vi "Get Debugger.vi"(8 "error in (no error)":errorcluster, 11 "Main In":refnum<class "Main.lvclass">) -> (0 "error out":errorcluster, 2 "Debugger.lvclass":refnum<class "Debugger.lvclass">, 3 "Main Out":refnum<class "Main.lvclass">)   [LabVIEW 2020, in "Main.lvclass"]
uses:
  Main.lvclass
  Debugger/Debugger.lvclass
  Main.lvclass/Main.ctl
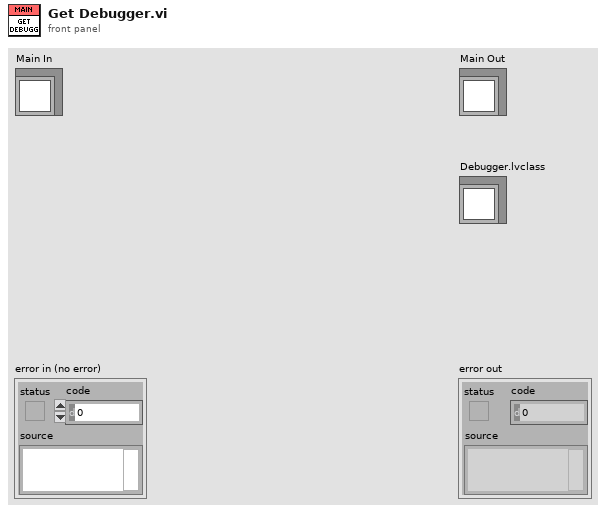
[diagram p1: front panel]
types:
  T1 = map{string, refnum<class "Debug Process.lvclass">}
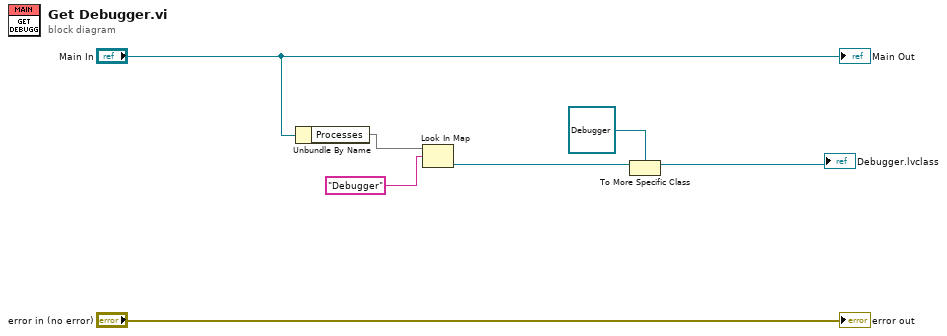
[diagram p0: block diagram]
diagram:
  n1 = Unbundle By Name("Main In") -> ("Processes"=w5:T1)
  n2 = Look In Map(map=w5, key="Debugger" ("Name")) -> (value=w3:refnum<class "Debug Process.lvclass">)  [unwired: 1 in, 1 out]
  n3 = To More Specific Class(target class=refnum<class "Debugger.lvclass"> refnum ("Debugger.lvclass"), reference=w3) -> (specific class reference=→"Debugger.lvclass":refnum<class "Debugger.lvclass">)  [unwired: 1 in, 1 out]
  "error out" <- "error in (no error)"
  "Main Out" <- "Main In"
